vi "Database Command Execute.vi"(8 "error in (no error)":errorcluster caption="错误输入（无错误）", 11 "Database Command 输入":refnum<class "Database Command.lvclass"> caption="DNL_LabVIEW Object in") -> (0 "error out":errorcluster caption="错误输出", 1 "Database Recordset.lvclass":refnum<class "Database Recordset.lvclass">, 3 "Database Command 输出":refnum<class "Database Command.lvclass"> caption="DNL_LabVIEW Object out")   [LabVIEW 2011, in "Database Command.lvclass"]
uses:
  Database Command.lvclass
  Recordset/Database Recordset.lvclass
  Database Command.lvclass/Database Command.ctl
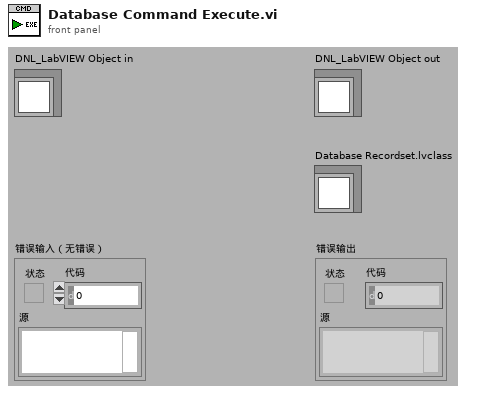
[diagram p1: front panel]
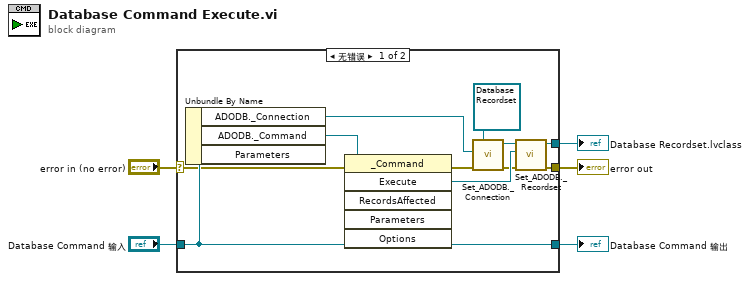
[diagram p0: block diagram]
diagram:
  n1 = case shown="无错误" "error in (no error)" {
    selector: "error in (no error)" -> [w14 w18]
    tunnel: [w11 w18] -> w4
    tunnel: [w16 w17] -> w2
    tunnel: "Database Command 输入" -> [w16 w17]
    tunnel: [w12 _] -> w1
    frame No Error {
      n2 = Unbundle By Name(w16) -> ("ADODB._Connection"=w10:refnum<k7>, "ADODB._Command"=w15:refnum<k7>)  [unwired: 1 out]
      n3 = invoke class="_Command" method="Execute"(reference=w15, error in=w14) -> (error out=w7:errorcluster, "Execute"=w13:refnum<k7>)  [unwired: 4 in, 4 out]
      n4 = call "Set_ADODB._Connection.vi"("error in (no error)"=w7, "ADODB._Connection"=w10, "Database Recordset输入"=refnum<class "Database Recordset.lvclass"> refnum ("Database Recordset.lvclass")) -> ("error out"=w6:errorcluster, "Database Recordset输出"=w8:refnum<class "Database Recordset.lvclass">)  [unwired: 7 in]
      n5 = call "Set_ADODB._Recordset.vi"("error in (no error)"=w6, "ADODB._Recordset"=w13, "Database Recordset输入"=w8) -> ("error out"=w11:errorcluster, "Database Recordset输出"=w12:refnum<class "Database Recordset.lvclass">)  [unwired: 7 in]
    }
    frame Error {
    }
  }
  "error out" <- w4
  "Database Command 输出" <- w2
  "Database Recordset.lvclass" <- w1
